vi "Get Channel Data and Trigger.vi"(4 "Channel Offsets":T1=[0, 0, 0, 0], 6 "Produce Dummy Data":bool, 7 "Invert Channels":bool, 8 "Stop Trigger Terminal":T2, 9 "Advance Trigger Terminal":T2, 10 "Period Trigger Terminal":T2, 11 "Acquisition Trigger Terminal":T2) -> (0 "Raw Data":T1, 1 "Overvoltage":bool, 2 "Trigger Signals":T3, 3 "Data":T1)   [LabVIEW 2014]
uses:
  Multi-Channel Analog Input Data.ctl
  Trigger Input Terminals.ctl
  Trigger Signals.ctl
  <vilib>/rvi/eio/common/nirviEmuTemplateMethod_errors.vi
  <vilib>/eio/EIONode/EIONode.xnode
panel:
  out "Data Valid":bool
  # "Copyright 2014 Vidrio Technologies\nScanImage 5 software is licensed under the Apache License, Version 2.0 (the \"License\"); you may not use any files contained\nwithin the ScanImage 5 release except in compliance with the License. You may obtain a copy of the License at\n http://www.apache.org/licenses/LICENSE-2.0\nUnless required by applicable law or agreed to in writing, software distributed under the License is distributed on an\n\"AS IS\" BASIS, WITHOUT WARRANTIES OR CONDITIONS OF ANY KIND, either express or implied. See the License for the\n specific language governing permissions and limitations under the License."
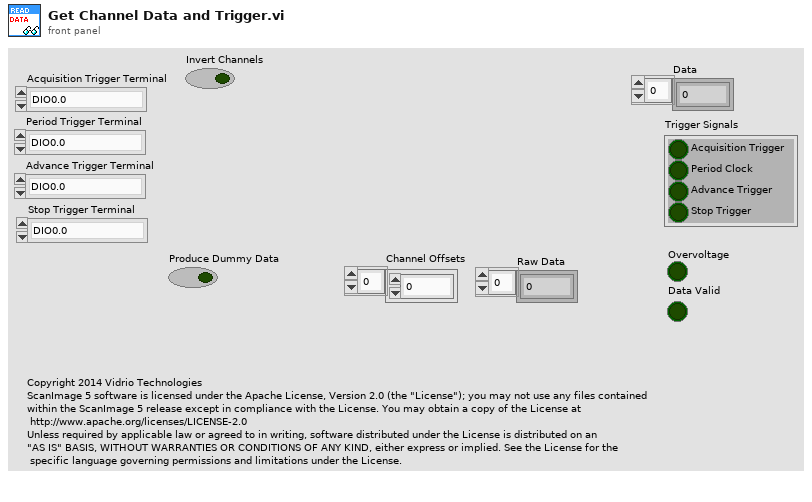
[diagram p1: front panel]
types:
  T1 = typedef "Multi-Channel Analog Input Data.ctl" = i16[]
  T2 = typedef "Trigger Input Terminals.ctl" = enum8{"DIO0.0", "DIO0.1", "DIO0.2", "DIO0.3", "PXI_Trig0", "PXI_Trig1", "PXI_Trig2", "PXI_Trig3", "PXI_Trig4", "PXI_Trig5", "PXI_Trig6", "PXI_Trig7", ""}
  T3 = typedef "Trigger Signals.ctl" = cluster{"Acquisition Trigger":bool, "Period Clock":bool, "Advance Trigger":bool, "Stop Trigger":bool}
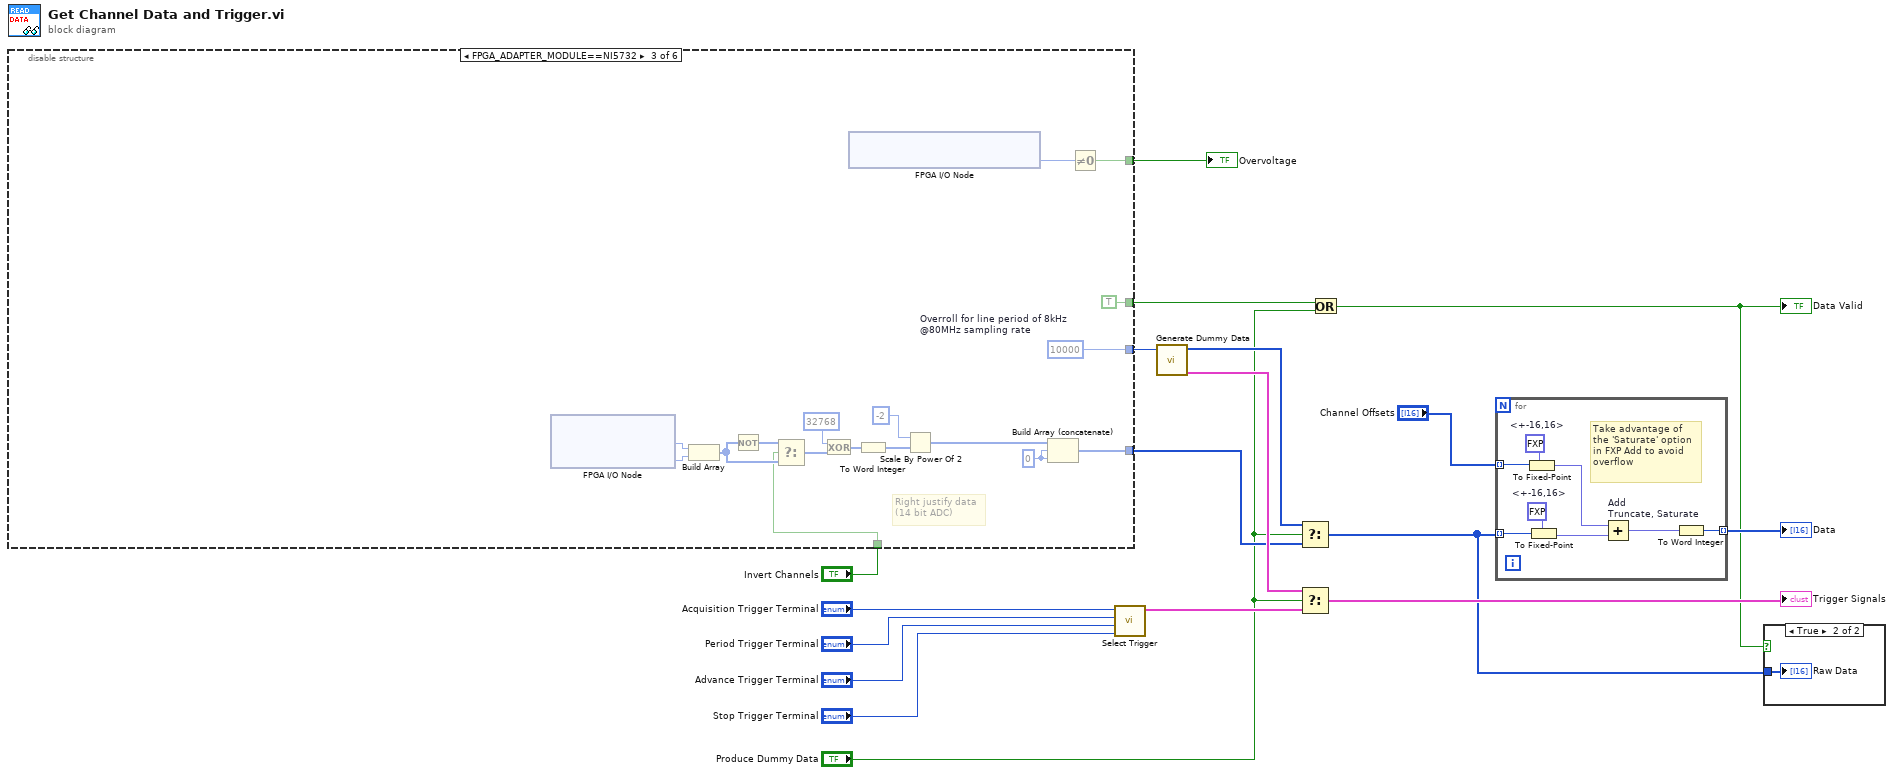
[diagram p0: block diagram]
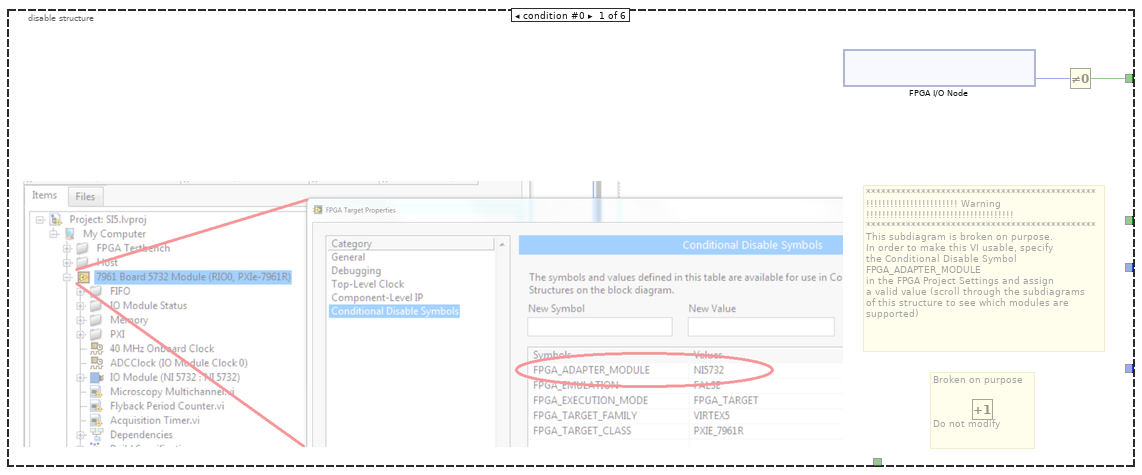
[diagram p3: hidden frame]
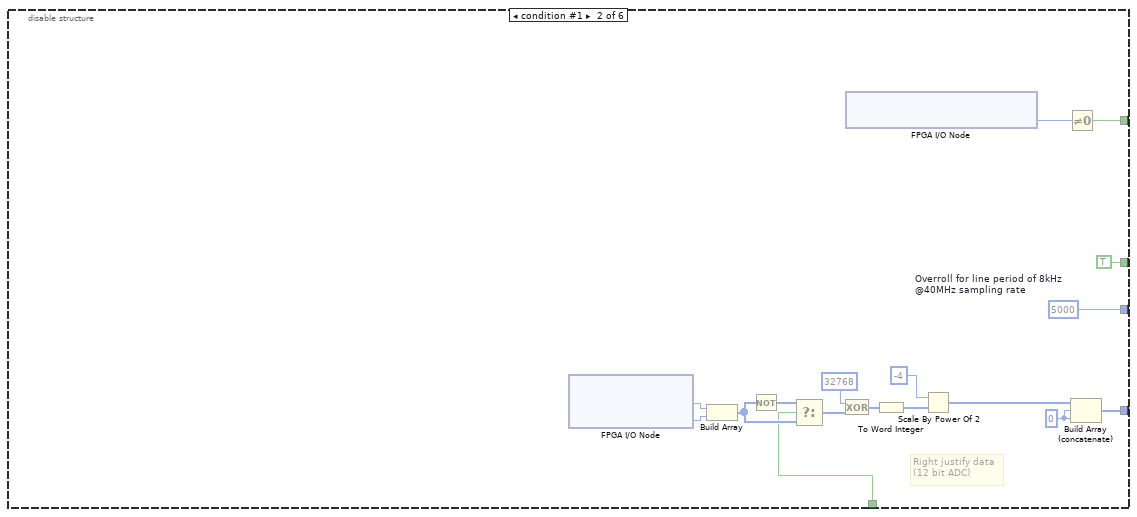
[diagram p4: hidden frame]
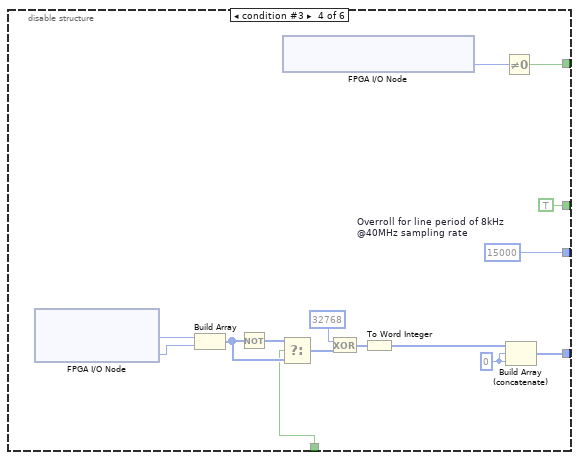
[diagram p5: hidden frame]
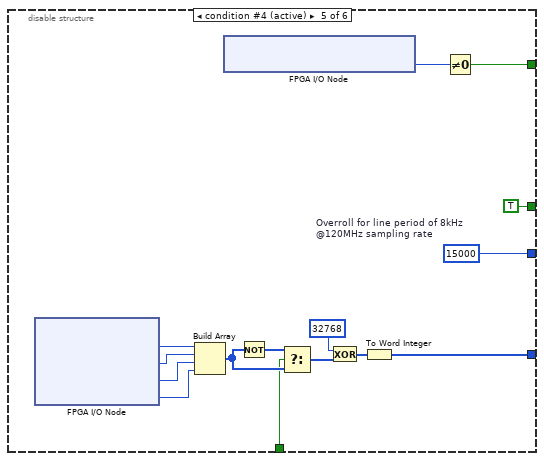
[diagram p6: hidden frame]
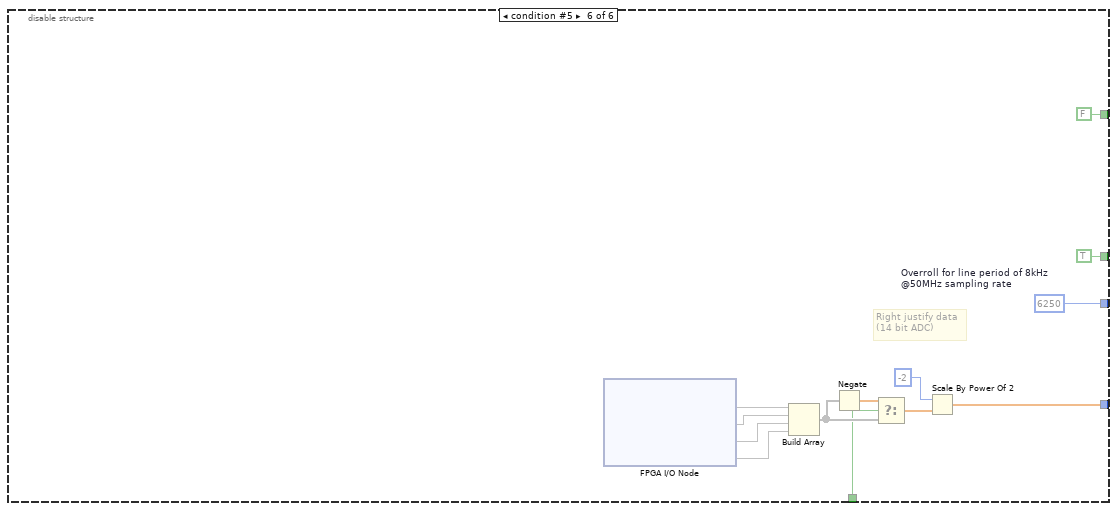
[diagram p7: hidden frame]
diagram:
  n1 = disable-structure shown="FPGA_ADAPTER_MODULE==NI5732" {
    disable-tunnel: [_ TRUE TRUE TRUE TRUE TRUE] -> w3
    disable-tunnel: "Invert Channels" -> [_ w25 w42 w61 w76 w85]
    disable-tunnel: [_ w24 w41 w58 w75 w95] -> w6
    disable-tunnel: [_ w23 w40 w57 w74 w93] -> w5
    disable-tunnel: [w19 w21 w38 w55 w70 FALSE ("Overvoltage")] -> w4
    frame condition #0 {
      # "**********************************************\n!!!!!!!!!!!!!!!!!!!!!!! Warning !!!!!!!!!!!!!!!!!!!!!!!!!!!!!!!!!!!!!\n**********************************************\nThis subdiagram is broken on purpose.\nIn order to make this VI usable, specify\nthe Conditional Disable Symbol\nFPGA_ADAPTER_MODULE\nin the FPGA Project Settings and assign\na valid value (scroll through the subdiagrams\nof this structure to see which modules are\nsupported)"
      # "Broken on purpose\n\n\n\nDo not modify"
      n2 = xnode "FPGA I/O Node"() -> ("IO Module\\DC Over Voltage"=w20:u8)  [unwired: 1 in, 1 out]
      n3 = Increment() -> ()  [unwired: 1 in, 1 out]
      n4 = Not Equal To 0?(x=w20) -> (x != 0?=w19:bool)
    }
    frame condition #1 {
      w32 = i16 0 ("16bit integer")
      w24 = i16 5000  # Overroll for line period of 8kHz @40MHz sampling rate
      # "Right justify data\n(12 bit ADC)"
      n5 = xnode "FPGA I/O Node"() -> ("IO Module\\AI 0"=w36:u16, "IO Module\\AI 1"=w35:u16)  [unwired: 2 in, 2 out]
      n6 = Build Array(w36, w35) -> (w27:u16[])
      n7 = Not(x=w27) -> (.not. x?=w28:u16[])
      n8 = Select(t=w28, s=w25, f=w27) -> (s? t:f=w26:u16[])
      n9 = Exclusive Or(1:w26, 2:u16 32768 ("x")) -> (0:w30:u16[])
      n10 = xnode "FPGA I/O Node"() -> ("IO Module\\DC Over Voltage"=w22:u8)  [unwired: 1 in, 1 out]
      n11 = To Word Integer(number=w30) -> (16bit integer=w31:i16[])
      n12 = Scale By Power Of 2(n=i16 -4, x=w31) -> (x*2^n=w33:i16[])
      n13 = Not Equal To 0?(x=w22) -> (x != 0?=w21:bool)
      n14 = Build Array (concatenate)(w33, w32, w32) -> (w23:i16[])
    }
    frame condition #2 {
      w49 = i16 0 ("16bit integer")
      w41 = i16 10000  # Overroll for line period of 8kHz @80MHz sampling rate
      # "Right justify data\n(14 bit ADC)"
      n15 = xnode "FPGA I/O Node"() -> ("IO Module\\AI 0"=w53:u16, "IO Module\\AI 1"=w52:u16)  [unwired: 2 in, 2 out]
      n16 = Build Array(w53, w52) -> (w44:u16[])
      n17 = Not(x=w44) -> (.not. x?=w45:u16[])
      n18 = Select(t=w45, s=w42, f=w44) -> (s? t:f=w43:u16[])
      n19 = Exclusive Or(1:w43, 2:u16 32768 ("x")) -> (0:w47:u16[])
      n20 = xnode "FPGA I/O Node"() -> ("IO Module\\DC Over Voltage"=w39:u8)  [unwired: 1 in, 1 out]
      n21 = To Word Integer(number=w47) -> (16bit integer=w48:i16[])
      n22 = Scale By Power Of 2(n=i16 -2, x=w48) -> (x*2^n=w50:i16[])
      n23 = Build Array (concatenate)(w50, w49, w49) -> (w40:i16[])
      n24 = Not Equal To 0?(x=w39) -> (x != 0?=w38:bool)
    }
    frame condition #3 {
      w60 = i16 0 ("16bit integer")
      w58 = i16 15000  # Overroll for line period of 8kHz @40MHz sampling rate
      n25 = xnode "FPGA I/O Node"() -> ("IO Module\\AI 0"=w63:u16, "IO Module\\AI 1"=w62:u16)  [unwired: 2 in, 2 out]
      n26 = Build Array(w63, w62) -> (w65:u16[])
      n27 = Not(x=w65) -> (.not. x?=w66:u16[])
      n28 = Select(t=w66, s=w61, f=w65) -> (s? t:f=w64:u16[])
      n29 = xnode "FPGA I/O Node"() -> ("IO Module\\DC Over Voltage"=w56:u8)  [unwired: 1 in, 1 out]
      n30 = Exclusive Or(1:w64, 2:u16 32768 ("x")) -> (0:w68:u16[])
      n31 = To Word Integer(number=w68) -> (16bit integer=w59:i16[])
      n32 = Not Equal To 0?(x=w56) -> (x != 0?=w55:bool)
      n33 = Build Array (concatenate)(w59, w60, w60) -> (w57:i16[])
    }
    frame condition #4 (active) {
      w75 = i16 15000  # Overroll for line period of 8kHz @120MHz sampling rate
      n34 = xnode "FPGA I/O Node"() -> ("IO Module\\AI 0"=w78:u16, "IO Module\\AI 1"=w77:u16, "IO Module\\AI 2"=w73:u16, "IO Module\\AI 3"=w72:u16)  [unwired: 4 in, 4 out]
      n35 = Build Array(w78, w77, w73, w72) -> (w80:u16[])
      n36 = xnode "FPGA I/O Node"() -> ("IO Module\\DC Over Voltage"=w71:u8)  [unwired: 1 in, 1 out]
      n37 = Not(x=w80) -> (.not. x?=w81:u16[])
      n38 = Select(t=w81, s=w76, f=w80) -> (s? t:f=w79:u16[])
      n39 = Exclusive Or(1:w79, 2:u16 32768 ("x")) -> (0:w83:u16[])
      n40 = To Word Integer(number=w83) -> (16bit integer=w74:i16[])
      n41 = Not Equal To 0?(x=w71) -> (x != 0?=w70:bool)
    }
    frame condition #5 {
      w95 = i16 6250  # Overroll for line period of 8kHz @50MHz sampling rate
      # "Right justify data\n(14 bit ADC)"
      n42 = xnode "FPGA I/O Node"() -> ("IO Module\\AI A0"=w92, "IO Module\\AI A1"=w91, "IO Module\\AI A2"=w90, "IO Module\\AI A3"=w89)  [unwired: 4 in, 4 out]
      n43 = Build Array(w92, w91, w90, w89) -> (w86:void[])
      n44 = Negate(x=w86) -> (-x=w87:dbl[])
      n45 = Select(t=w87, s=w85, f=w86) -> (s? t:f=w88:dbl[])
      n46 = Scale By Power Of 2(n=i16 -2, x=w88) -> (x*2^n=w93:dbl[])
    }
  }
  "Overvoltage" <- w4
  n47 = call "Select Trigger.vi"("Stop Trigger Terminal"="Stop Trigger Terminal", "Advance Trigger Terminal"="Advance Trigger Terminal", "Period Trigger Terminal"="Period Trigger Terminal", "Acquisition Trigger Terminal"="Acquisition Trigger Terminal") -> ("Trigger Signals"=w15:T3)  [unwired: 7 in]
  n48 = call "Generate Dummy Data.vi"("Overroll"=w6) -> ("Trigger"=w14:T3, "Data"=w13:i16[])  [unwired: 9 in]
  n49 = Select(t=w13, s="Produce Dummy Data", f=w5) -> (s? t:f=w8:i16[])
  n50 = Select(t=w14, s="Produce Dummy Data", f=w15) -> (s? t:f=→"Trigger Signals":T3)
  n51 = Or(x=w3, y="Produce Dummy Data") -> (x .or. y?=w1:bool)
  "Data Valid" <- w1
  n52 = for {
    tunnel: w8 -> [w105] mode=indexing
    tunnel: "Channel Offsets" -> [w101] mode=indexing
    tunnel: [w98] -> w9 mode=indexing
    w102 = fxp<+/-,16,16> 0.0  # <+-16,16>
    w104 = fxp<+/-,16,16> 0.0  # <+-16,16>
    # "Take advantage of\nthe 'Saturate' option\nin FXP Add to avoid\noverflow"
    n53 = To Fixed-Point(fixed-point type=w102, number=w101) -> (fixed-point=w100:fxp<+/-,16,16>)
    n54 = To Fixed-Point(fixed-point type=w104, number=w105) -> (fixed-point=w103:fxp<+/-,16,16>)
    n55 = Add "Add\nTruncate, Saturate"(x=w100, y=w103) -> (x+y=w99:fxp<+/-,16,16>)
    n56 = To Word Integer(number=w99) -> (16bit integer=w98:i16)
  }
  "Data" <- w9
  n57 = case shown="True" w1 {
    tunnel: w8 -> [_ w106]
    frame False {
    }
    frame True {
      "Raw Data" <- w106
    }
  }
